vi "Create.vi"(5 "Server Fixture in":refnum<class "Server Fixture.lvclass">, 8 "error in (no error)":errorcluster) -> (0 "error out":errorcluster, 3 "Server Fixture":refnum<class "Server Fixture.lvclass">)   [LabVIEW 2013, in "libssh2_integration_tests.lvlib" / "Server Fixture.lvclass"]
uses:
  Server Fixture.lvclass
  Server Fixture.lvclass/Server Fixture.ctl
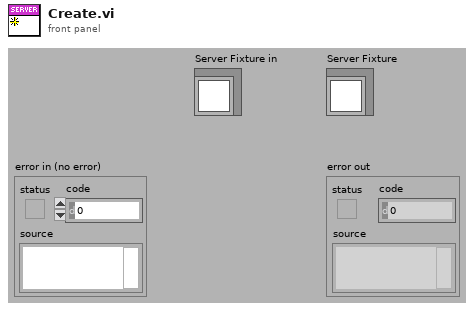
[diagram p1: front panel]
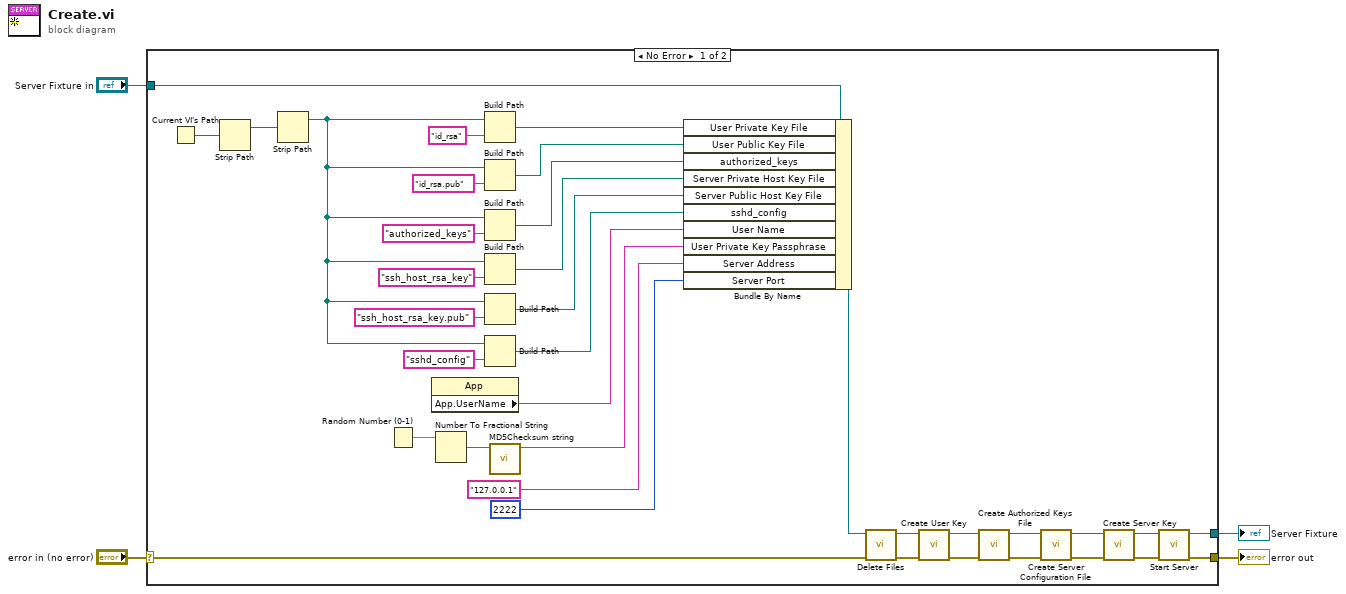
[diagram p0: block diagram]
diagram:
  n1 = case shown="No Error" "error in (no error)" {
    selector: "error in (no error)" -> [w20 w42]
    tunnel: [w12 w42] -> w3
    tunnel: [w10 w41] -> w1
    tunnel: "Server Fixture in" -> [w40 w41]
    frame No Error {
      n2 = Current VI's Path() -> (path=w38:path)
      n3 = Strip Path(path=w38) -> (stripped path=w22:path)  [unwired: 1 out]
      n4 = Strip Path(path=w22) -> (stripped path=w21:path)  [unwired: 1 out]
      n5 = Random Number (0-1)() -> (number: 0 to 1=w31:dbl)
      n6 = property class="App"() -> ("App.UserName"=w32:string)  [unwired: 2 in, 2 out]
      n7 = Number To Fractional String(number=w31) -> (F-format string=w30:string)  [unwired: 3 in]
      n8 = Build Path(base path=w21, name or relative path="id_rsa") -> (appended path=w35:path)
      n9 = Build Path(base path=w21, name or relative path="id_rsa.pub") -> (appended path=w34:path)
      n10 = Build Path(base path=w21, name or relative path="authorized_keys") -> (appended path=w33:path)
      n11 = Build Path(base path=w21, name or relative path="ssh_host_rsa_key") -> (appended path=w27:path)
      n12 = Build Path(base path=w21, name or relative path="ssh_host_rsa_key.pub") -> (appended path=w24:path)
      n13 = Build Path(base path=w21, name or relative path="sshd_config") -> (appended path=w26:path)
      n14 = call <vilib>:"MD5Checksum string.vi"("Message String"=w30) -> ("MD5 message-digest"=w23:string)  [unwired: 10 in]
      n15 = Bundle By Name(cluster=w40, "User Private Key File"=w35, "User Public Key File"=w34, "authorized_keys"=w33, "Server Private Host Key File"=w27, "Server Public Host Key File"=w24, "sshd_config"=w26, "User Name"=w32, "User Private Key Passphrase"=w23, "Server Address"="127.0.0.1", "Server Port"=u16 2222) -> (w5:refnum<class "Server Fixture.lvclass">)
      n16 = call "Delete Files.vi"("error in (no error)"=w20, "Server Fixture in"=w5) -> ("error out"=w7:errorcluster, "Server Fixture out"=w6:refnum<class "Server Fixture.lvclass">)  [unwired: 8 in]
      n17 = call "Create User Key.vi"("error in (no error)"=w7, "Server Fixture in"=w6) -> ("error out"=w19:errorcluster, "Server Fixture out"=w17:refnum<class "Server Fixture.lvclass">)  [unwired: 8 in]
      n18 = call "Create Authorized Keys File.vi"("error in (no error)"=w19, "Server Fixture in"=w17) -> ("error out"=w18:errorcluster, "Server Fixture out"=w15:refnum<class "Server Fixture.lvclass">)  [unwired: 8 in]
      n19 = call "Create Server Configuration File.vi"("error in (no error)"=w18, "Server Fixture in"=w15) -> ("error out"=w16:errorcluster, "Server Fixture out"=w13:refnum<class "Server Fixture.lvclass">)  [unwired: 8 in]
      n20 = call "Create Server Key.vi"("error in (no error)"=w16, "Server Fixture in"=w13) -> ("error out"=w14:errorcluster, "Server Fixture out"=w11:refnum<class "Server Fixture.lvclass">)  [unwired: 8 in]
      n21 = call "Start Server.vi"("error in (no error)"=w14, "Server Fixture in"=w11) -> ("error out"=w12:errorcluster, "Server Fixture out"=w10:refnum<class "Server Fixture.lvclass">)  [unwired: 8 in]
    }
    frame Error {
    }
  }
  "error out" <- w3
  "Server Fixture" <- w1
